vi "applyNewTimes.vi"(8 "error in (no error)":errorcluster, 11 "ScriptEventList in":refnum<class "ScriptEventList.lvclass">) -> (0 "error out":errorcluster, 3 "ScriptEventList out":refnum<class "ScriptEventList.lvclass">)   [LabVIEW 2009, in "Tools.lvlib" / "Scripting.lvlib" / "ScriptEventList.lvclass"]
uses:
  ScriptEventList.lvclass
  ScriptEventList.lvclass/ScriptEventList.ctl
  ScriptEvent.lvclass
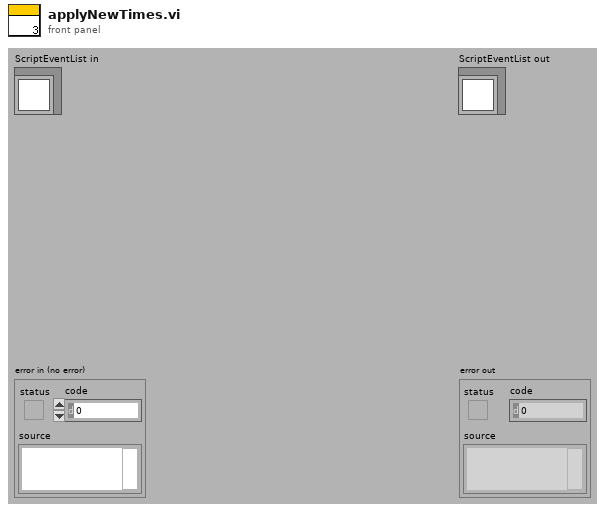
[diagram p1: front panel]
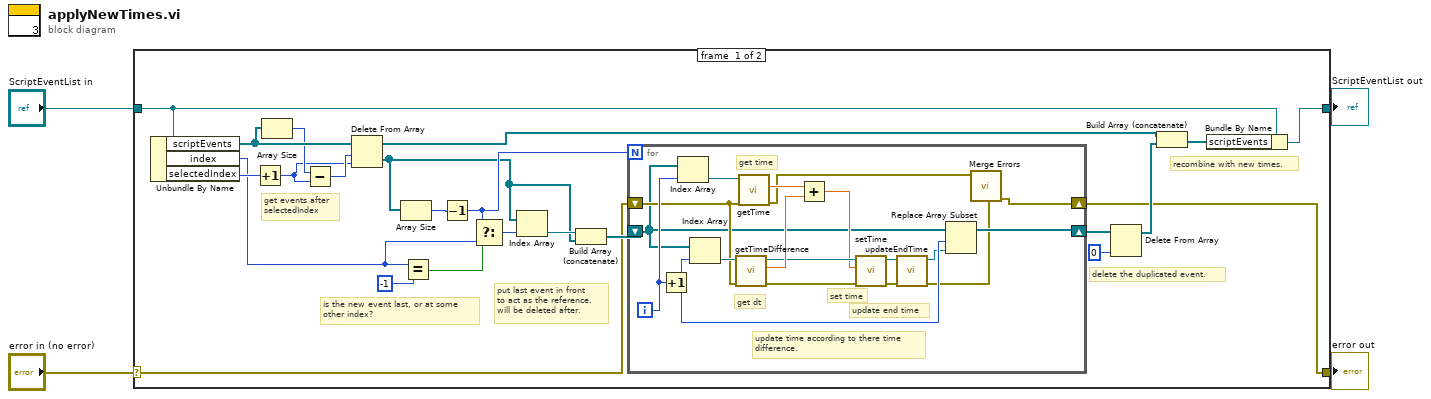
[diagram p0: block diagram]
diagram:
  n1 = case shown="No Error" "error in (no error)" {
    selector: "error in (no error)" -> [w17 w47]
    tunnel: [w9 w47] -> w3
    tunnel: [w10 w46] -> w1
    tunnel: "ScriptEventList in" -> [w11 w46]
    frame #0 {
      # "is the new event last, or at some \nother index?"
      # "recombine with new times."
      # "delete the duplicated event."
      # "put last event in front\nto act as the reference.\nwill be deleted after."
      # "get events after\nselectedIndex"
      n2 = Unbundle By Name(w11) -> ("scriptEvents"=w27:refnum<class "ScriptEvent.lvclass">[], "index"=w5:i32, "selectedIndex"=w26:i32)
      n3 = Increment(x=w26) -> (x+1=w7:i32)
      n4 = Array Size(array=w27) -> (size(s)=w8:i32)
      n5 = Subtract(x=w8, y=w7) -> (x-y=w25:i32)
      n6 = Delete From Array(array=w27, length=w25, index=w7) -> (deleted portion=w6:refnum<class "ScriptEvent.lvclass">[], array with subset deleted=w14:refnum<class "ScriptEvent.lvclass">[])
      n7 = Array Size(array=w6) -> (size(s)=w21:i32)
      n8 = Equal?(x=w5, y=-1) -> (x = y?=w24:bool)
      n9 = Decrement(x=w21) -> (x-1=w20:i32)
      n10 = Select(t=w20, s=w24, f=w5) -> (s? t:f=w23:i32)
      n11 = Index Array(array=w6, index=w23) -> (element=w19:refnum<class "ScriptEvent.lvclass">)
      n12 = Build Array (concatenate)(w19, w6) -> (w18:refnum<class "ScriptEvent.lvclass">[])
      n13 = for {
        N: w20 -> [_]
        shift-right: [w34] -> w16
        shift-left: w18 -> [w36]
        shift-right: [w32] -> w9
        shift-left: w17 -> [w42]
        i -> [w45]
        # "update end time"
        # "update time according to there time \ndifference."
        # "get time"
        # "set time"
        # "get dt"
        n14 = Increment(x=w45) -> (x+1=w35:i32)
        n15 = Index Array(array=w36, index=w45) -> (element=w44:refnum<class "ScriptEvent.lvclass">)
        n16 = Index Array(array=w36, index=w35) -> (element=w43:refnum<class "ScriptEvent.lvclass">)
        n17 = call "getTimeDifference.vi"("error in (no error)"=w42, "ScriptEvent.lvclass in"=w43) -> ("error out"=w37:errorcluster, "time difference"=w40:dbl, "ScriptEvent.lvclass out"=w39:refnum<class "ScriptEvent.lvclass">)  [unwired: 7 in]
        n18 = call "getTime.vi"("error in (no error)"=w42, "ScriptEvent.lvclass in"=w44) -> ("error out"=w33:errorcluster, "time"=w41:dbl)  [unwired: 7 in, 1 out]
        n19 = Add(x=w41, y=w40) -> (x+y=w38:dbl)
        n20 = call "setTime.vi"("error in (no error)"=w37, "time"=w38, "ScriptEvent.lvclass in"=w39) -> ("error out"=w31:errorcluster, "ScriptEvent.lvclass out"=w30:refnum<class "ScriptEvent.lvclass">)  [unwired: 7 in]
        n21 = call-dynamic "updateEndTime.vi"("error in (no error)"=w31, "ScriptEvent in"=w30) -> ("error out"=w28:errorcluster, "ScriptEvent out"=w29:refnum<class "ScriptEvent.lvclass">)  [unwired: 8 in]
        n22 = Replace Array Subset(array=w36, new element=w29, index=w35) -> (w34:refnum<class "ScriptEvent.lvclass">[])
        n23 = call <vilib>:"Merge Errors.vi"("error in 2 (no error)"=w28, "error in 1 (no error)"=w33) -> ("error out"=w32:errorcluster)  [unwired: 5 in]
      }
      n24 = Delete From Array(array=w16, index=0) -> (array with subset deleted=w13:refnum<class "ScriptEvent.lvclass">[])  [unwired: 1 in, 1 out]
      n25 = Build Array (concatenate)(w14, w13) -> (w12:refnum<class "ScriptEvent.lvclass">[])
      n26 = Bundle By Name(cluster=w11, "scriptEvents"=w12) -> (w10:refnum<class "ScriptEventList.lvclass">)
    }
    frame #1 {
    }
  }
  "error out" <- w3
  "ScriptEventList out" <- w1
